vi "SPC_set_mode.vi"(6 "Modul Type to Simulate":T1 items=["Hardware Modus"=0, "SPC-600 Simulation"=600, "SPC-630 Simulation"=630, "SPC-700  Simulation"=700, "SPC-730  Simulation"=730, "SPC-130  Simulation"=130, "SPC-830  Simulation"=830, "SPC-140  Simulation"=140, "SPC-930  Simulation"=930, "DPC-230  Simulation"=230, "SPC-150  Simulation"=150, "SPC-150 N  Simulation"=151, "SPC-150 NX  Simulation"=152, "SPC-130 EM  Simulation"=131, "SPC-130 EMN  Simulation"=132, "SPC-130 IN Simulation"=135, "SPC-130 INX Simulation"=136, "SPC-130 INXX Simulation"=137, "SPC-160  Simulation"=160, "SPC-160 X  Simulation"=161, "SPC-160 PCIE  Simulation"=162, "SPC-180 Simulation"=180, "SPC-181 Simulation"=181, "SPC-182 Simulation"=182, "SPC-185 Simulation"=185, "SPC-186 Simulation"=186, "SPC-187 Simulation"=187, "DPC-330  Simulation"=330, "DPC-590  Simulation"=590, "TDC-104 Simulation"=104], 7 "Force Use":bool, 8 "Error In":errorcluster, 11 "DLL Path":path) -> (0 "Error Out":errorcluster, 3 "DLL Path":path)   [LabVIEW 2019]
doc: "Input parameters:\nmode mode of DLL operation\nforce_use force using the module if they are locked ( in use)\n*in_use pointer to the table with information which module must be used\nReturn value: on success - DLL mode, on error <0 (error code)\nThe procedure is used to change the mode of the DLL operation between the hardware mode \nand the simulation mode. It is also used to switch the DLL to the simulation mode if hardware \nerrors occur during the initialisation.\nTable ‘in_use’ should contain entries for all 8 modules:\n0 – means that the module will be unlocked and not used longer\n1 – means that the module will be initialised and locked\nWhen the Hardware Mode is requested for each of 8 possible modules:\n-if ‘in_use’ entry = 1 : the proper module is locked and initialised (if it wasn’t) with the \ninitial parameters set (from ini_file) but only when it was not locked by another \napplication or when ‘force_use’ = 1.\n-if ‘in_use’ entry = 0 : the proper module is unlocked and cannot be used further.\nWhen one of the simulation modes is requested for each of 8 possible modules:\n-if ‘in_use’ entry = 1 : the proper module is initialised (if it wasn’t) with the initial \nparameters set (from ini_file).\n-if ‘in_use’ entry = 0 : the proper module is unlocked and cannot be used further.\nErrors during the module initialisation can cause that the module is excluded from use.\nUse the function SPC_get_init_status and/or SPC_get_module_info to check which modules \nare correctly initialised and can be use further.\nUse the function SPC_get_mode to check which mode is actually set. Possible ‘mode’ values \nare defined in the spcm_def.h file.\n\ninfo@becker-hickl.com"
uses:
  SPC_Controls/ModuleTypes.ctl
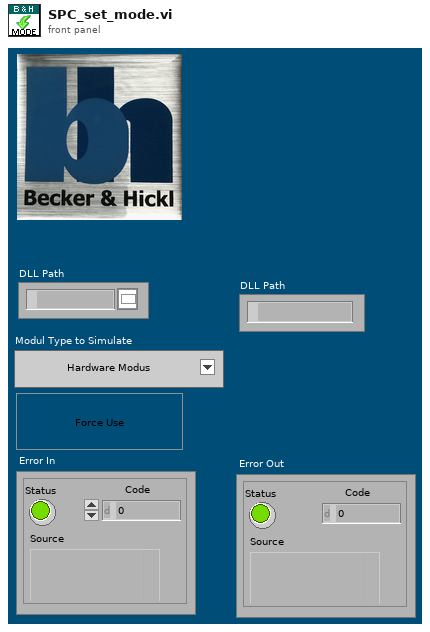
[diagram p1: front panel]
types:
  T1 = typedef "ModuleTypes.ctl" = i16
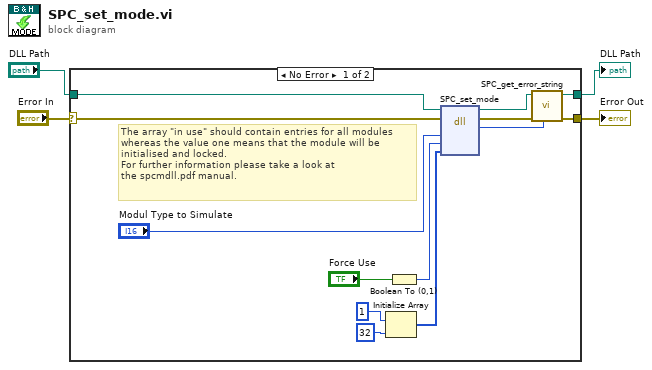
[diagram p0: block diagram]
diagram:
  n1 = case shown="No Error" "Error In" {
    selector: "Error In" -> [w16 w19]
    tunnel: "DLL Path" -> [w17 w18]
    tunnel: [w12 w19] -> w3
    tunnel: [w11 w18] -> w2
    frame No Error {
      # "The array \"in use\" should contain entries for all modules\nwhereas the value one means that the module will be\ninitialised and locked.\nFor further information please take a look at \nthe spcmdll.pdf manual."
      n2 = Initialize Array(1, 32) -> (w7:i32[])
      n3 = Boolean To (0,1)(Boolean="Force Use") -> (0, 1=w15:i16)
      n4 = dll-call lib="D:/spcm/lib/lab_view/lv10.0/spcm32.dll" fn="SPC_set_mode"(path in=w17, error in=w16, "mode"="Modul Type to Simulate", "force_use"=w15, "in_use"=w7) -> (path out=w14:path, error out=w13:errorcluster, "return type"=w10:i16)  [unwired: 4 in]
      n5 = call "SPC_get_error_string.vi"("ErrorID"=w10, "Error In"=w13, "DLL Path"=w14) -> ("Error Out"=w12:errorcluster, "DLL Path"=w11:path)  [unwired: 6 in, 1 out]
    }
    frame Error {
    }
  }
  "Error Out" <- w3
  "DLL Path" <- w2
